vi "mt.vi"() -> ()   [LabVIEW 2022 SP3]
panel:
  out "数组":string[][](array[string])
  in  "停止":bool
  in  "确定按钮":bool
  in  "布尔":bool
  in  "数值":dbl
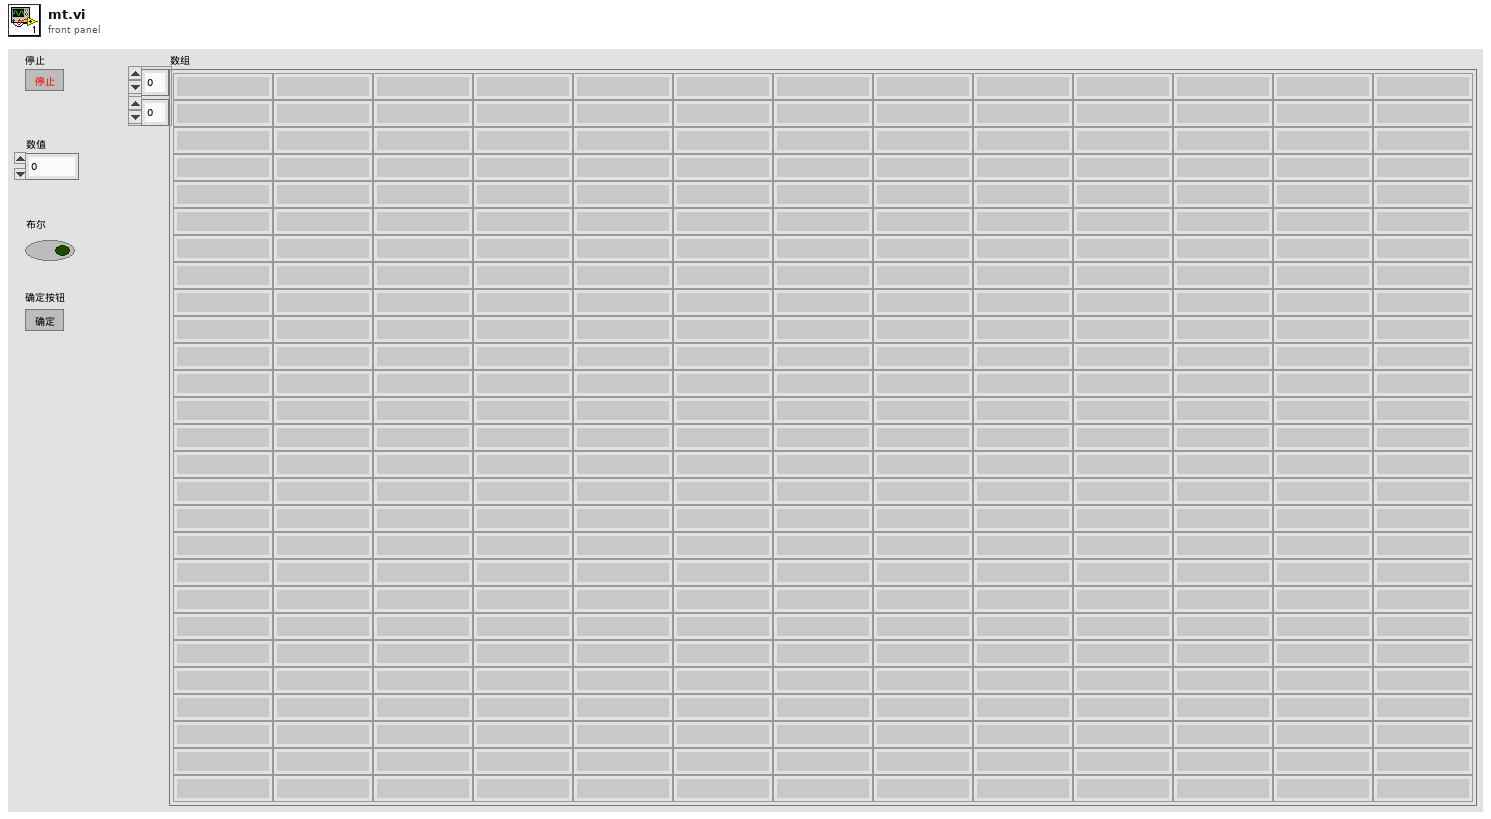
[diagram p1: front panel]
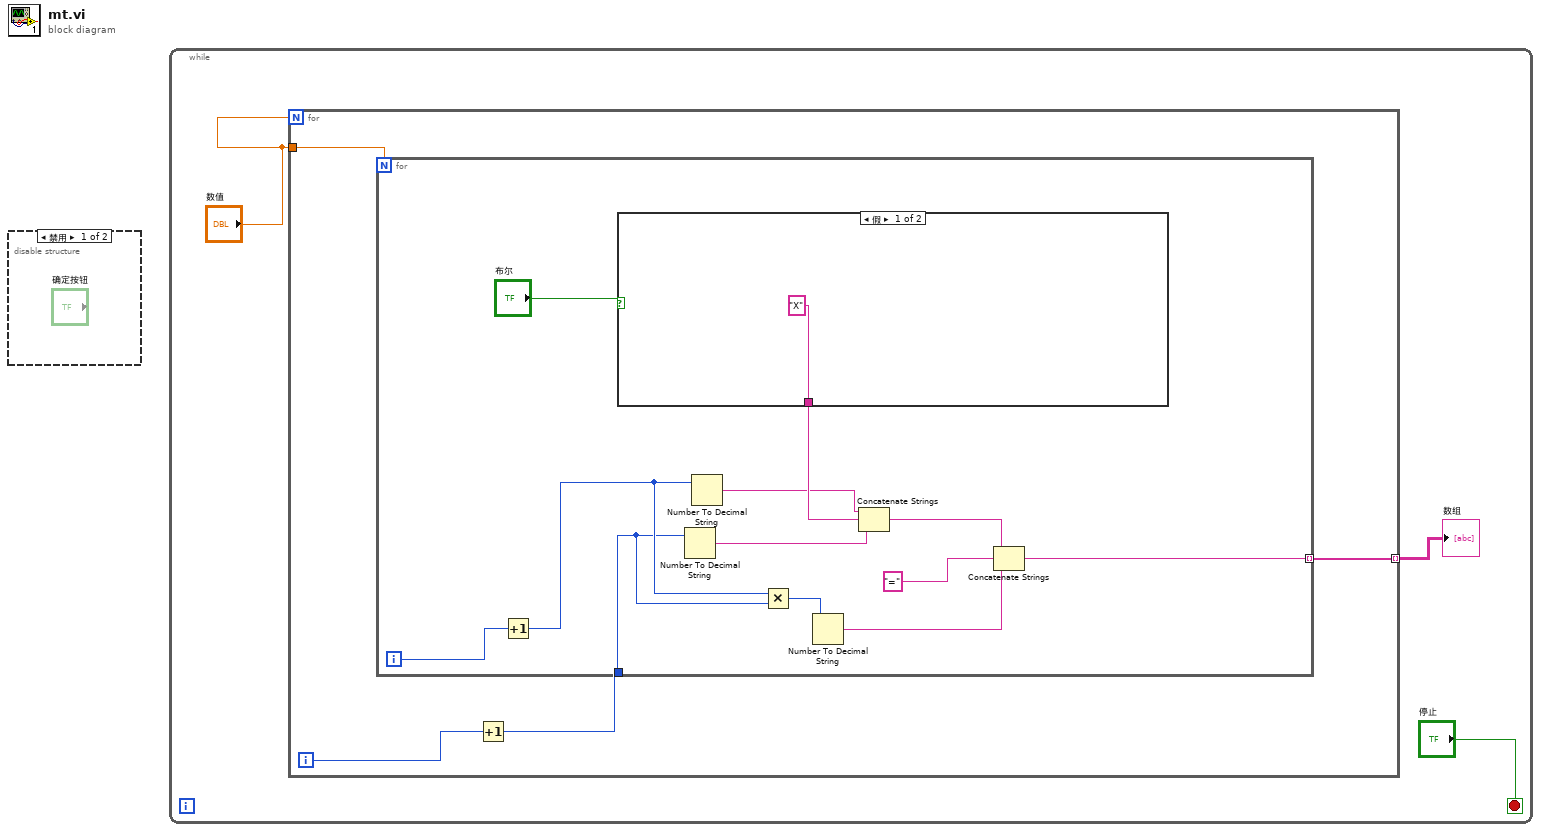
[diagram p0: block diagram]
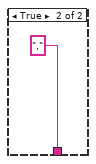
[diagram p3: hidden frame]
diagram:
  n1 = disable-structure shown="禁用" {
    frame Disabled {
    }
    frame Enabled {
    }
  }
  n2 = while {
    stop <- "停止" stop-if-true
    n3 = for {
      N: "数值" -> [_]
      tunnel: "数值" -> [w7]
      tunnel: [w4] -> w2 mode=indexing
      i -> [w6]
      n4 = Increment(x=w6) -> (x+1=w5:i32)
      n5 = for {
        N: w7 -> [_]
        tunnel: w5 -> [w16]
        tunnel: [w8] -> w4 mode=indexing
        i -> [w18]
        n6 = Increment(x=w18) -> (x+1=w17:i32)
        n7 = case shown="假" "布尔" {
          tunnel: ["X" ","] -> w15
          frame False {
          }
          frame True {
          }
        }
        n8 = Number To Decimal String(number=w16) -> (decimal integer string=w13:string)  [unwired: 1 in]
        n9 = Number To Decimal String(number=w17) -> (decimal integer string=w14:string)  [unwired: 1 in]
        n10 = Multiply(x=w17, y=w16) -> (x*y=w10:i32)
        n11 = Number To Decimal String(number=w10) -> (decimal integer string=w9:string)  [unwired: 1 in]
        n12 = Concatenate Strings(w14, w15, w13) -> (w11:string)
        n13 = Concatenate Strings(w11, "=" ("字符串"), w9) -> (w8:string)
      }
    }
    "数组" <- w2
  }
